vi "Read Default Value.vi"(8 "error in (no error)":errorcluster, 11 "Path Data Type in":refnum<class "Path Data Type.lvclass">) -> (0 "error out":errorcluster, 2 "Default Value":string, 3 "Path Data Type out":refnum<class "Path Data Type.lvclass">)   [LabVIEW 2018, in "Path Data Type.lvclass"]
uses:
  Path Data Type.lvclass
  Path Data Type.lvclass/Path Data Type.ctl
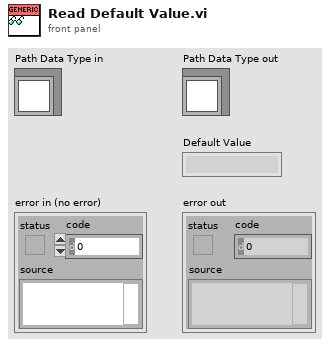
[diagram p1: front panel]
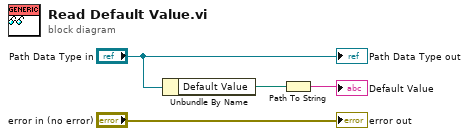
[diagram p0: block diagram]
diagram:
  n1 = Unbundle By Name("Path Data Type in") -> ("Default Value"=w2:path)
  n2 = Path To String(path=w2) -> (string=→"Default Value":string)
  "error out" <- "error in (no error)"
  "Path Data Type out" <- "Path Data Type in"
